vi "NavigatorInputPrimitive.vi"(0 "error in":errorcluster, 2 "Component":T2, 3 "node":string) -> (1 "error out":errorcluster, 4 "Navigator Inputs":T1)   [LabVIEW 2012]
doc: "This VI gets the status of the Navigator Buttons"
uses:
  <userlib>/ROS for LabVIEW Software/ROS/Code/SubVIs/BaxterButtons.ctl
  <userlib>/ROS for LabVIEW Software/ROS/Code/Console/Servers/ServerSubs/TopicDef.ctl
  <userlib>/ROS for LabVIEW Software/ROS/Code/SubVIs/_ROSDirection.ctl
panel:
  out "Reply":string
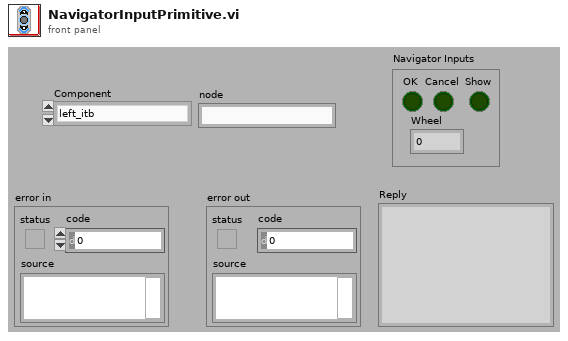
[diagram p1: front panel]
types:
  T1 = cluster{"OK":bool, "Cancel":bool, "Show":bool, "Wheel":u8}
  T2 = typedef "BaxterButtons.ctl" = enum16{"left_itb", "right_itb", "torso_left_itb", "torso_right_itb"}
  T3 = typedef "TopicDef.ctl" = cluster{"Topic":string, "Type":string, "Action":T4, "Update (ms)":u16, "queue size":u16}
  T4 = typedef "_ROSDirection.ctl" = enum16{"Node", "Publisher", "Subscriber", "ServiceClient", "ServiceProvider"}
  T5 = typedef "_ROSControl.ctl" = cluster{"topic port":u16, "Node":string, "topic":string, "type":string, "node port":u16, "error ":errorcluster, "Direction":T4, "Update (ms)":u16, "FIFO size":u16}
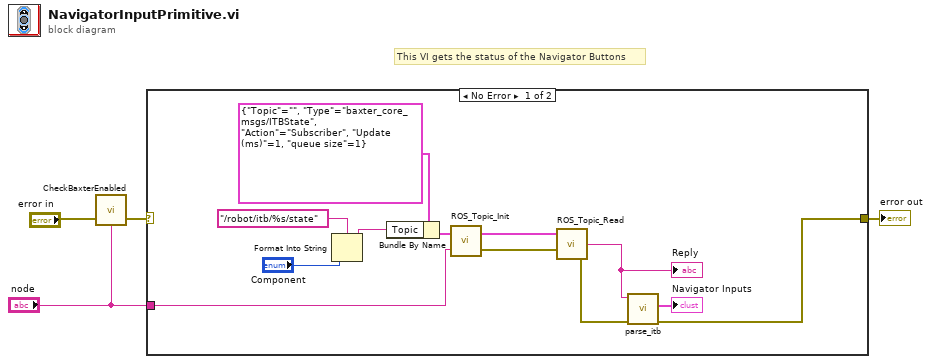
[diagram p0: block diagram]
diagram:
  # "This VI gets the status of the Navigator Buttons"
  n1 = call <userlib>:"CheckBaxterEnabled.vi"("error in"="error in", "node"="node") -> ("error out"=w2:errorcluster)  [unwired: 2 in]
  n2 = case shown="No Error" w2 {
    selector: w2 -> [_ w17]
    tunnel: [w5 w17] -> w4
    tunnel: "node" -> [w8 _]
    frame No Error {
      n3 = Format Into String(format string="/robot/itb/%s/state" ("topic"), "Component") -> (resulting string=w13:string)  [unwired: 2 in, 1 out]
      n4 = Bundle By Name(cluster=T3 {"Topic"="", "Type"="baxter_core_msgs/ITBState", "Action"=enum."Subscriber", "Update (ms)"=1, "queue size"=1} ("Definitions"), "Topic"=w13) -> (w9:T3)
      n5 = call <userlib>:"ROS_Topic_Init.vi"("node"=w8, "Definitions"=w9) -> ("error out"=w6:errorcluster, "ROS out"=w16:T5)
      n6 = call <userlib>:"ROS_Topic_Read.vi"("error in (no error)"=w6, "ROS in"=w16) -> ("error out"=w7:errorcluster, "Reply"=w15:string)  [unwired: 1 in, 1 out]
      "Reply" <- w15
      n7 = call <userlib>:"parse_itb.vi"("error in"=w7, "msg in"=w15) -> ("error out"=w5:errorcluster, "Navigator Inputs"=→"Navigator Inputs":T1)  [unwired: 3 in, 1 out]
    }
    frame Error {
    }
  }
  "error out" <- w4
